vi "Allan Variance for range.vi"(8 "error in (no error)":errorcluster, 9 "Frequency":dbl=115.0 format="%#_13g", 10 "n range":i32, 11 "Data in":dbl[](array[numeric])) -> (0 "error out":errorcluster, 2 "Allan Variances":dbl[][](array[numeric]), 3 "Allan Variances graph":cluster{dbl[], dbl[]}(graph))   [LabVIEW 2021]
uses:
  IMU Processing.lvlib
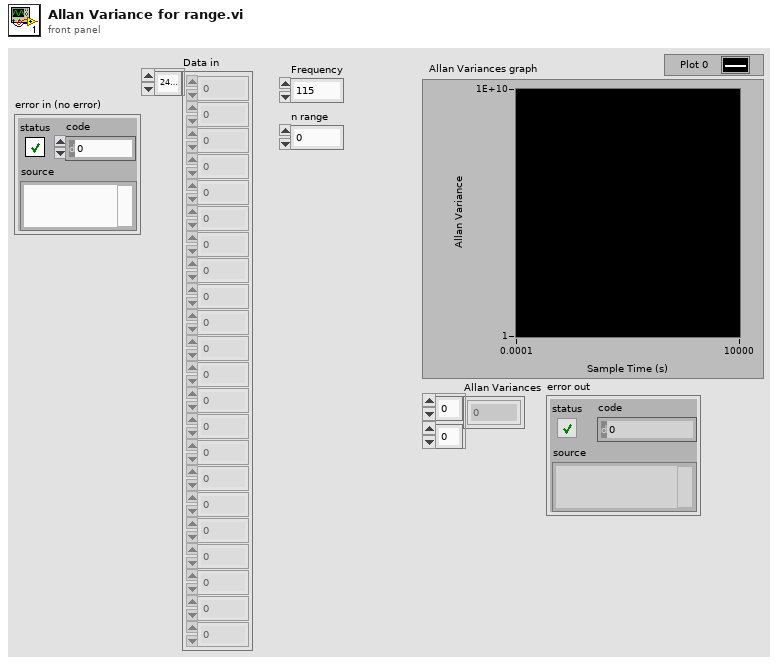
[diagram p1: front panel]
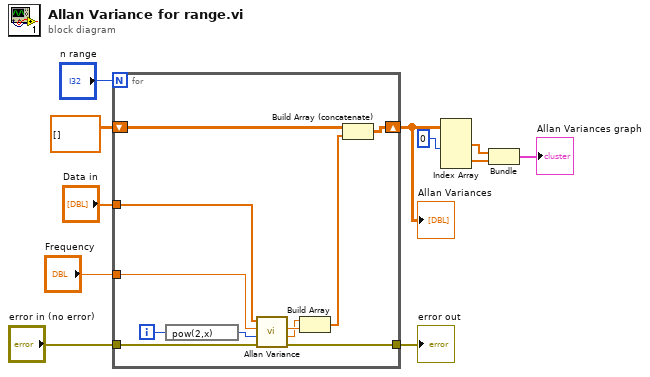
[diagram p0: block diagram]
diagram:
  n1 = for {
    N: "n range" -> [_]
    shift-right: [w22] -> w9
    shift-left: dbl[][] [] -> [w21]
    tunnel: "Frequency" -> [w19]
    tunnel: [w18] -> w3
    tunnel: "error in (no error)" -> [w13]
    tunnel: "Data in" -> [w12]
    i -> [w16]
    n2 = expression code="pow(2,x)"(w16) -> (w15:i32)
    n3 = call "Allan Variance.vi"("error in (no error)"=w13, "n"=w15, "Frequency (Hz)"=w19, "Data in"=w12) -> ("error out"=w18:errorcluster, "actual sample time (s)"=w14:dbl, "Allan Variance"=w17:dbl)  [unwired: 5 in]
    n4 = Build Array(w14, w17) -> (w20:dbl[])
    n5 = Build Array (concatenate)(w21, w20) -> (w22:dbl[][])
  }
  "Allan Variances" <- w9
  "error out" <- w3
  n6 = Index Array(array=w9, index (col) #1=0 ("disabled index (col)")) -> (element #1=w7:dbl[], element #2=w6:dbl[])  [unwired: 3 in]
  n7 = Bundle(w7, w6) -> (→"Allan Variances graph":cluster{dbl[], dbl[]})  [unwired: 1 in]
